vi "Create Common Input Controls.vi"(0 "Common DistanceLimitAnchor":dbl=150.0, 1 "Common Input AnchorArray":refnum<class "Anchor.lvclass">[](array[class]), 5 "Common Position Estimation Method":u32(ring) caption="Position Estimation Method" items=["Star Configuration", "Swarm Method"], 7 "Common Max V variatie":dbl=10.0 format="%#_13g", 9 "Common Max h variatie":dbl=30.0 format="%#_13g", 11 "Common Enable error margin":bool=TRUE, 12 "Common Error margin":i32=2) -> (8 "Common Input Cluster":T1={"Common Input AnchorArray"=[], "Common DistanceLimitAnchor"=150.0, "Common Position Estimation Method"=0, "Common Max V variatie"=10.0, "Common Max h variatie"=30.0, "Common Enable error margin"=TRUE, "Common Error margin"=2} {"Common Max h variatie" format="%#_13g"; "Common Max V variatie" format="%#_13g"; "Common Position Estimation Method" items=["Star Configuration", "Swarm Method"]})   [LabVIEW 2014]
doc: "This VI creates all common input controls necessary for both star-configuration and swarm method position estimation algorithms. This information is clustered so it will take less space as input, which results in more readable source code."
uses:
  Anchor/Anchor.lvclass
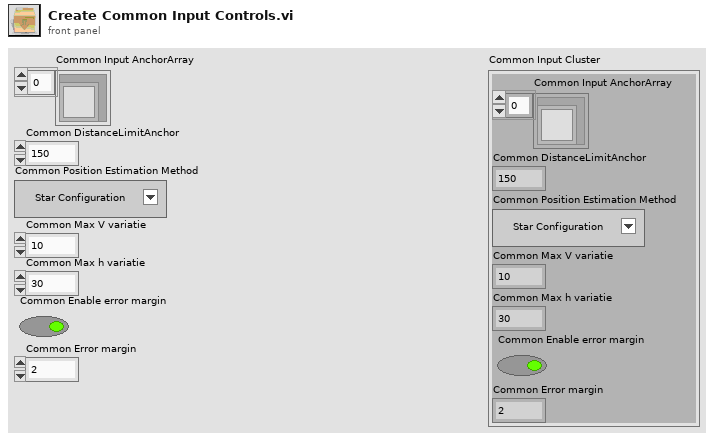
[diagram p1: front panel]
types:
  T1 = cluster{"Common Input AnchorArray":refnum<class "Anchor.lvclass">[], "Common DistanceLimitAnchor":dbl, "Common Position Estimation Method":u32, "Common Max V variatie":dbl, "Common Max h variatie":dbl, "Common Enable error margin":bool, "Common Error margin":i32}
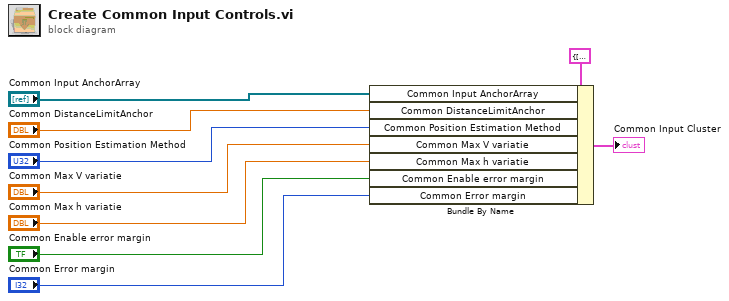
[diagram p0: block diagram]
diagram:
  n1 = Bundle By Name(cluster=T1 {"Common Input AnchorArray"=[refnum, refnum, refnum], "Common DistanceLimitAnchor"=150.0, "Common Position Estimation Method"=0, "Common Max V variatie"=10.0, "Common Max h variatie"=30.0, "Common Enable error margin"=FALSE, "Common Error margin"=2} ("Common Input Cluster 2"), "Common Input AnchorArray"="Common Input AnchorArray", "Common DistanceLimitAnchor"="Common DistanceLimitAnchor", "Common Position Estimation Method"="Common Position Estimation Method", "Common Max V variatie"="Common Max V variatie", "Common Max h variatie"="Common Max h variatie", "Common Enable error margin"="Common Enable error margin", "Common Error margin"="Common Error margin") -> (→"Common Input Cluster":T1)
